vi "tm451_dcimgrecorder_wmetadata.vi"() -> ()   [LabVIEW 2021]
panel:
  out "Frames Recorded":i32
  in  "DCIMG Path":path
  in  "Frames":i32=100
  out "Error Out":errorcluster
  # "This is an example of how to use the\nhard disk recorder functions to record\nimages to a DCIMG file and how to\nwrite metadata to the file."
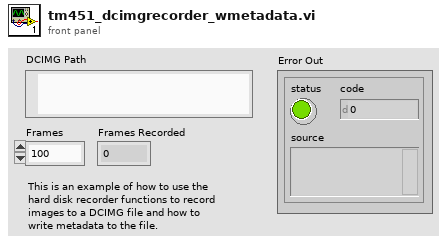
[diagram p1: front panel]
types:
  T1 = cluster{"Model":string, "Camera ID":string, "Firmware":string}
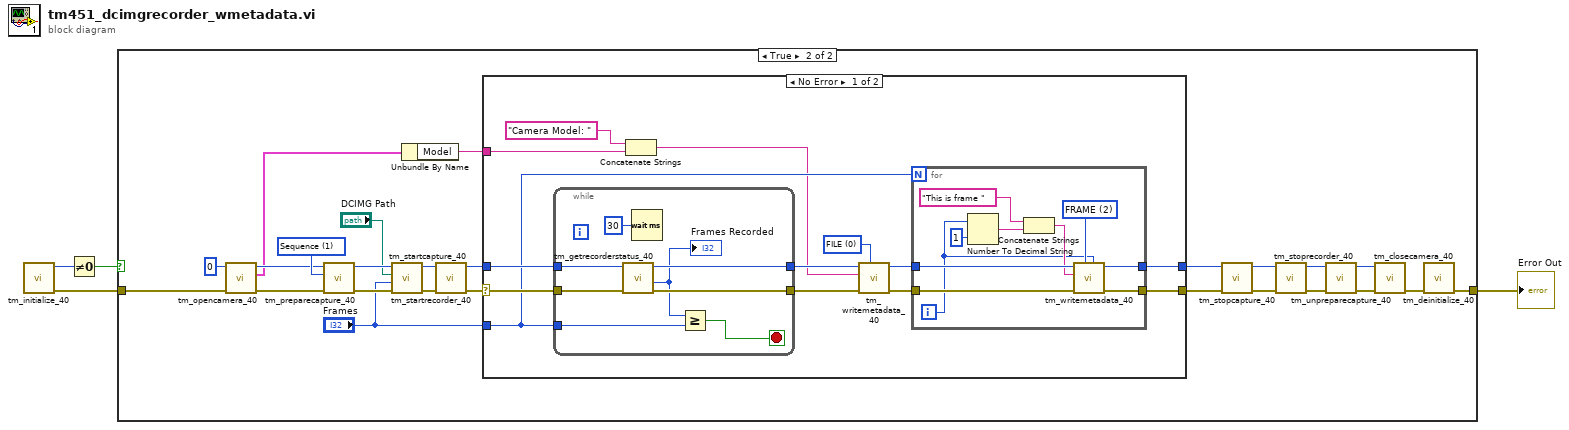
[diagram p0: block diagram]
diagram:
  n1 = call <userlib>:"tm_initialize_40.vi"() -> ("error out"=w1:errorcluster, "Number Of Cameras"=w2:u32)  [unwired: 8 in, 2 out]
  n2 = Not Equal To 0?(x=w2) -> (x != 0?=w4:bool)
  n3 = case shown="True" w4 {
    tunnel: w1 -> [w5 w30]
    tunnel: [w5 w26] -> w3
    frame False {
    }
    frame True {
      w28 = 1 items=["Snap", "Sequence"] ("Capture mode")
      n4 = call <userlib>:"tm_opencamera_40.vi"("error in (no error)"=w30, "Camera Index"=u32 0) -> ("error out"=w14:errorcluster, "Camera Details"=w13:T1, "Handle out"=w15:u32)  [unwired: 7 in]
      n5 = call <userlib>:"tm_preparecapture_40.vi"("error in (no error)"=w14, "Capture mode"=w28, "Handle in"=w15) -> ("error out"=w23:errorcluster, "Handle out"=w22:u32)  [unwired: 5 in, 2 out]
      n6 = call <userlib>:"tm_startrecorder_40.vi"("error in (no error)"=w23, "frames"="Frames", "File"="DCIMG Path", "Handle in"=w22) -> ("error out"=w21:errorcluster, "Handle out"=w20:u32)  [unwired: 6 in]
      n7 = Unbundle By Name(w13) -> ("Model"=w12:string)
      n8 = call <userlib>:"tm_startcapture_40.vi"("error in (no error)"=w21, "Handle in"=w20) -> ("error out"=w19:errorcluster, "Handle out"=w18:u32)  [unwired: 8 in]
      n9 = case shown="No Error" w19 {
        selector: w19 -> [w43 w62]
        tunnel: w18 -> [w42 w63]
        tunnel: [w32 w63] -> w9
        tunnel: [w31 w62] -> w8
        tunnel: "Frames" -> [w41 _]
        tunnel: w12 -> [w34 _]
        frame No Error {
          w36 = 0 items=["FILE"=0, "FRAME"=2] ("Type")
          n10 = while {
            tunnel: w43 -> [w59]
            tunnel: w42 -> [w58]
            tunnel: [w57] -> w37
            tunnel: [w60] -> w40
            tunnel: w41 -> [w61]
            stop <- w55 stop-if-true
            n11 = call <userlib>:"tm_getrecorderstatus_40.vi"("error in (no error)"=w59, "Handle"=w58) -> ("error out"=w57:errorcluster, "Count"=w56:i32, "Handle"=w60:u32)  [unwired: 6 in, 1 out]
            "Frames Recorded" <- w56
            n12 = Wait (ms)(milliseconds to wait=u32 30) -> ()  [unwired: 1 out]
            n13 = Greater Or Equal?(x=w56, y=w61) -> (x >= y?=w55:bool)
          }
          n14 = Concatenate Strings("Camera Model: ", w34) -> (w33:string)
          n15 = call <userlib>:"tm_writemetadata_40.vi"("Type"=w36, "error in (no error)"=w37, "Metadata"=w33, "Handle"=w40) -> ("error out"=w38:errorcluster, "Handle"=w39:u32)  [unwired: 6 in]
          n16 = for {
            N: w41 -> [_]
            tunnel: w38 -> [w52]
            tunnel: w39 -> [w53]
            tunnel: [w45] -> w32
            tunnel: [w44] -> w31
            i -> [w46]
            w48 = 2 items=["FILE"=0, "FRAME"=2] ("Type")
            n17 = Number To Decimal String(number=w46, width (-)=i16 1) -> (decimal integer string=w50:string)
            n18 = Concatenate Strings("This is frame ", w50) -> (w49:string)
            n19 = call <userlib>:"tm_writemetadata_40.vi"("Index"=w46, "Type"=w48, "error in (no error)"=w52, "Metadata"=w49, "Handle"=w53) -> ("error out"=w44:errorcluster, "Handle"=w45:u32)  [unwired: 5 in]
          }
        }
        frame Error {
        }
      }
      n20 = call <userlib>:"tm_stopcapture_40.vi"("error in (no error)"=w8, "Handle in"=w9) -> ("error out"=w6:errorcluster, "Handle out"=w7:u32)  [unwired: 8 in]
      n21 = call <userlib>:"tm_stoprecorder_40.vi"("error in (no error)"=w6, "Handle in"=w7) -> ("error out"=w10:errorcluster, "Handle out"=w11:u32)  [unwired: 8 in]
      n22 = call <userlib>:"tm_unpreparecapture_40.vi"("error in (no error)"=w10, "Handle in"=w11) -> ("error out"=w25:errorcluster, "Handle out"=w24:u32)  [unwired: 8 in]
      n23 = call <userlib>:"tm_closecamera_40.vi"("error in (no error)"=w25, "Handle in"=w24) -> ("error out"=w27:errorcluster)  [unwired: 9 in]
      n24 = call <userlib>:"tm_deinitialize_40.vi"("error in (no error)"=w27) -> ("error out"=w26:errorcluster)  [unwired: 10 in]
    }
  }
  "Error Out" <- w3
